vi "Received Data to Indicator Cluster.vi"(8 "Error In":errorcluster, 10 "Data":string) -> (0 "Error Out":errorcluster, 2 "output cluster":T1 {"Battery Level" scale=0.0..255.0})   [LabVIEW 2014]
uses:
  Controls/Controllers Clusters/Normal Operation Indicator Cluster.ctl
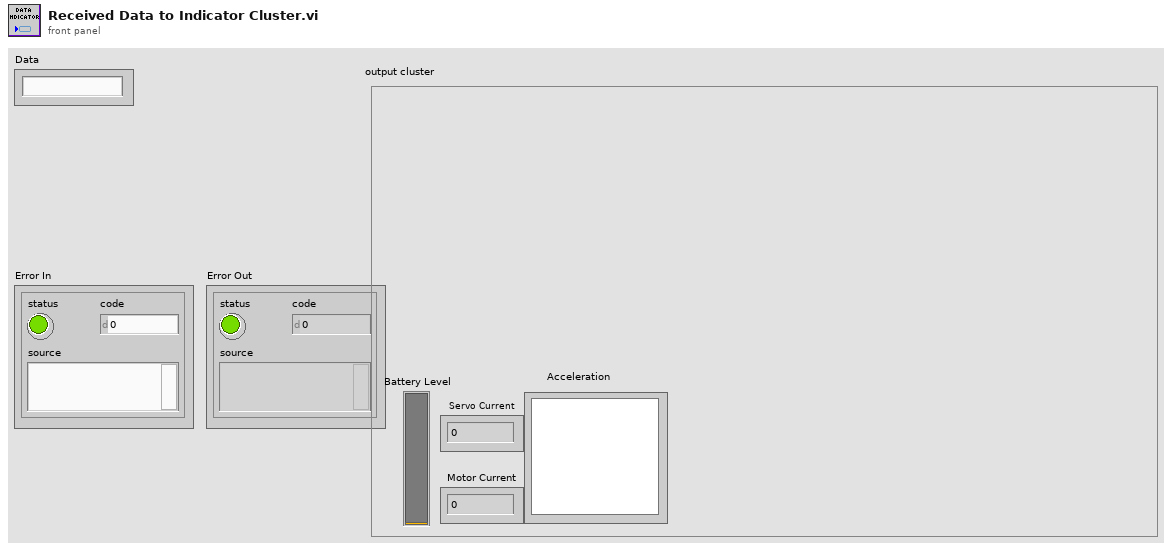
[diagram p1: front panel]
types:
  T1 = typedef "Normal Operation Indicator Cluster.ctl" = cluster{"Battery Level":u8, "Servo Current":dbl, "Motor Current":dbl, "Acceleration":cluster{"X":dbl, "Y":dbl}[]}
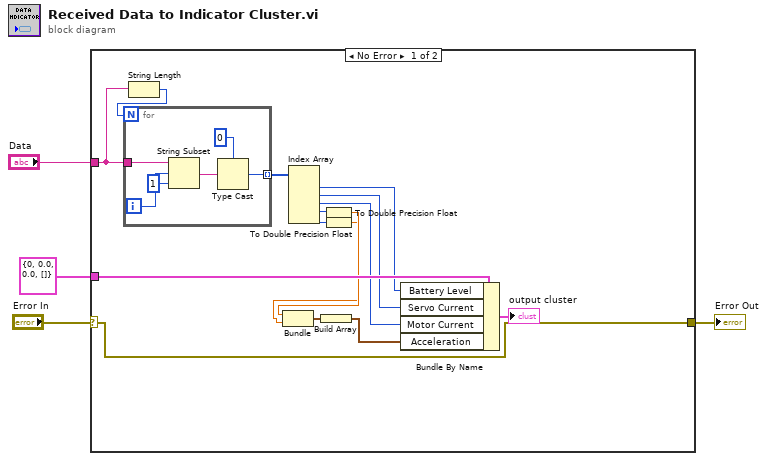
[diagram p0: block diagram]
diagram:
  n1 = case shown="No Error" "Error In" {
    selector: "Error In" -> [w8 w26]
    tunnel: [w8 w26] -> w3
    tunnel: "Data" -> [w6 _]
    tunnel: T1 {"Battery Level"=0, "Servo Current"=0.0, "Motor Current"=0.0, "Acceleration"=[]} ("Cluster") -> [w18 _]
    frame No Error {
      n2 = String Length(string=w6) -> (length=w5:i32)
      n3 = for {
        N: w5 -> [_]
        tunnel: w6 -> [w25]
        tunnel: [w20] -> w19 mode=indexing
        i -> [w24]
        n4 = String Subset(string=w25, offset (0)=w24, length (rest)=1 ("length (rest)")) -> (substring=w22:string)
        n5 = Type Cast(type=u8 0, x=w22) -> (*(type *) &x=w20:u8)
      }
      n6 = Index Array(array=w19) -> (element #1=w17:u8, element #2=w16:u8, element #3=w15:u8, element #4=w13:u8, element #5=w14:u8)  [unwired: 5 in]
      n7 = To Double Precision Float(number=w13) -> (double precision float=w12:dbl)
      n8 = To Double Precision Float(number=w14) -> (double precision float=w11:dbl)
      n9 = Bundle(w12, w11) -> (w10:cluster{dbl, dbl})  [unwired: 1 in]
      n10 = Build Array(w10) -> (w9:cluster{dbl, dbl}[])
      n11 = Bundle By Name(cluster=w18, "Battery Level"=w17, "Servo Current"=w16, "Motor Current"=w15, "Acceleration"=w9) -> (→"output cluster":T1)
    }
    frame Error {
    }
  }
  "Error Out" <- w3
